vi "Channel Handles Hierarchy to Channels Array.vi"(8 "error in":errorcluster, 11 "1553 channel handles":T2[](array[typedef]) {"terminal status channels" format="%.0x"; "messages"."Rx status handles" format="%.0x"; "messages"."Tx status handles" format="%.0x"; "messages"."timestamps" format="%.0x"; "messages"."parameters"."RxBC channel handle" format="%.0x"; "messages"."parameters"."RxRT channel handle" format="%.0x"; "messages"."parameters"."Tx channel handle" format="%.0x"}) -> (0 "error out":errorcluster, 2 "tx channels":T1[](array[typedef]) format="%.0x", 3 "rx channels":T1[](array[typedef]) format="%.0x")   [LabVIEW 2020, in "AIM MIL-STD-1553 Engine.lvlib" / "Implementation.lvlib" / "Execution Unit.lvclass"]
uses:
  Execution Unit.lvclass
  <vilib>/NI VeriStand/Custom Device API/Custom Device Item Ref.ctl
  <vilib>/NI VeriStand/Custom Device API/Custom Device API.lvlib
  Shared/1553 Channel Handles.ctl
  Parameter Handles.ctl
  Message Handles.ctl
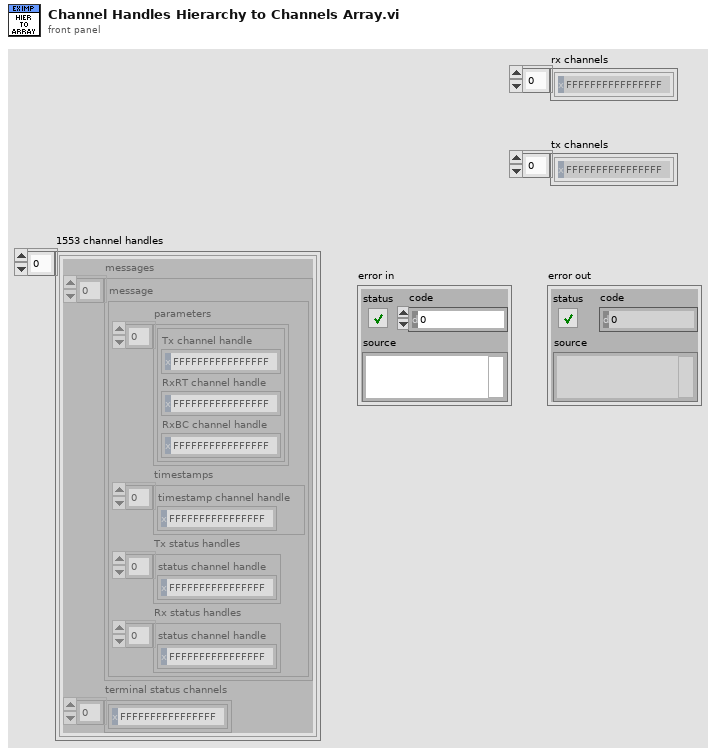
[diagram p1: front panel]
types:
  T1 = typedef "Custom Device API.lvlib/Custom Device Item Ref.ctl" = u64
  T2 = typedef "1553 Channel Handles.ctl" = cluster{"messages":T3[], "terminal status channels":T1[]}
  T3 = typedef "AIM MIL-STD-1553 Engine.lvlib/Implementation.lvlib/Execution Unit.lvclass/Message Handles.ctl" = cluster{"parameters":T4[], "timestamps":T1[], "Tx status handles":T1[], "Rx status handles":T1[]}
  T4 = typedef "AIM MIL-STD-1553 Engine.lvlib/Implementation.lvlib/Execution Unit.lvclass/Parameter Handles.ctl" = cluster{"Tx channel handle":T1, "RxRT channel handle":T1, "RxBC channel handle":T1}
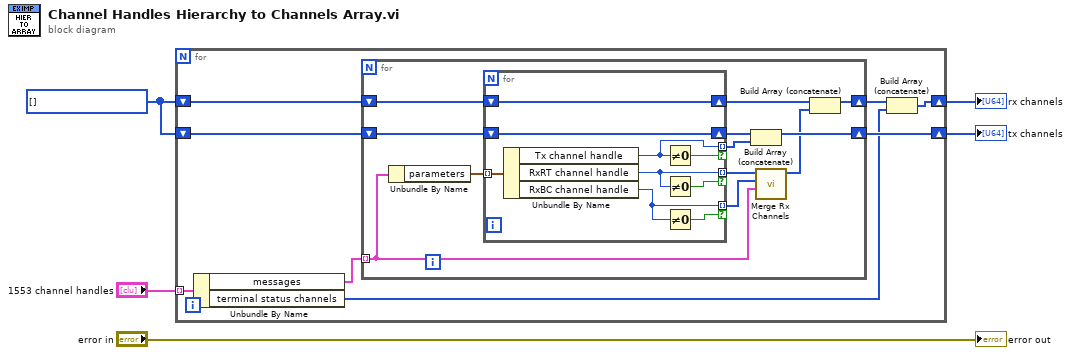
[diagram p0: block diagram]
diagram:
  w5 = T1[] [] ("Incoming Channels")
  n1 = for {
    tunnel: "1553 channel handles" -> [w13] mode=indexing
    shift-right: [w7] -> w2
    shift-left: w5 -> [w12]
    shift-right: [w10] -> w4
    shift-left: w5 -> [w11]
    n2 = Unbundle By Name(w13) -> ("messages"=w9:T3[], "terminal status channels"=w6:T1[])
    n3 = for {
      tunnel: w9 -> [w14] mode=indexing
      shift-right: [w21] -> w8
      shift-left: w12 -> [w25]
      shift-right: [w19] -> w10
      shift-left: w11 -> [w24]
      n4 = Unbundle By Name(w14) -> ("parameters"=w23:T4[])
      n5 = for {
        shift-right: [w33] -> w22
        shift-left: w25 -> [w33]
        tunnel: w23 -> [w34] mode=indexing
        shift-right: [w32] -> w20
        shift-left: w24 -> [w32]
        tunnel: [w29] -> w17 mode=indexing if=w30
        tunnel: [w28] -> w16 mode=indexing if=w27
        tunnel: [w26] -> w18 mode=indexing if=w31
        n6 = Unbundle By Name(w34) -> ("Tx channel handle"=w26:T1, "RxRT channel handle"=w29:T1, "RxBC channel handle"=w28:T1)
        n7 = Not Equal To 0?(x=w26) -> (x != 0?=w31:bool)
        n8 = Not Equal To 0?(x=w29) -> (x != 0?=w30:bool)
        n9 = Not Equal To 0?(x=w28) -> (x != 0?=w27:bool)
      }
      n10 = Build Array (concatenate)(w20, w18) -> (w19:T1[])
      n11 = call "Merge Rx Channels.vi"("message"=w14, "RxBC channel handles"=w16, "RxRT channel handles"=w17) -> ("Rx channel handles"=w15:T1[])  [unwired: 8 in]
      n12 = Build Array (concatenate)(w22, w15) -> (w21:T1[])
    }
    n13 = Build Array (concatenate)(w8, w6) -> (w7:T1[])
  }
  "rx channels" <- w2
  "tx channels" <- w4
  "error out" <- "error in"
